vi "doAction.vi"(8 "error in (no error)":errorcluster, 10 "ContextData":refnum<class "ContextData.lvclass">, 11 "Exit in":refnum<class "Exit.lvclass">) -> (0 "error out":errorcluster, 3 "Exit out":refnum<class "Exit.lvclass">)   [LabVIEW 2018, in "Exit.lvclass"]
uses:
  Exit.lvclass
  ContextData/ContextData.lvclass
  State/State.lvclass
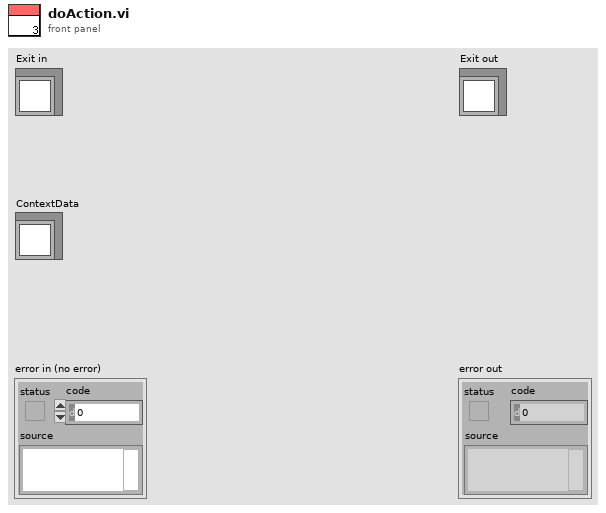
[diagram p1: front panel]
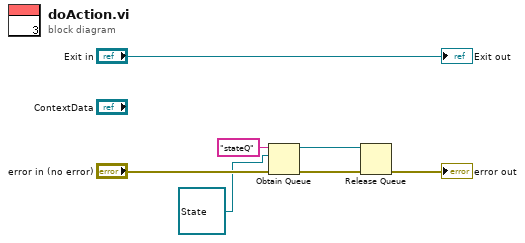
[diagram p0: block diagram]
diagram:
  n1 = Obtain Queue(name (unnamed)="stateQ", element data type=refnum<class "State.lvclass"> refnum ("State.lvclass"), error in (no error)="error in (no error)") -> (queue out=w1:refnum<queue>, error out=w5:errorcluster)  [unwired: 2 in, 1 out]
  n2 = Release Queue(queue=w1, error in (no error)=w5) -> (error out=→"error out":errorcluster)  [unwired: 1 in, 2 out]
  "Exit out" <- "Exit in"
